vi "get TextSummary.vi"(8 "error in (no error)":errorcluster, 11 "Category in":refnum<class "Category.lvclass">) -> (0 "error out":errorcluster, 2 "Text Summary":string, 3 "Category out":refnum<class "Category.lvclass">)   [LabVIEW 2013, in "Category.lvclass"]
doc: "Text Summary is the string that appears in the second column of the tree control. It summaries the state of the xceDataNode."
uses:
  Category.lvclass
  xCE/xceDataNode/xceDataNode.lvclass
  Category.lvclass/Category.ctl
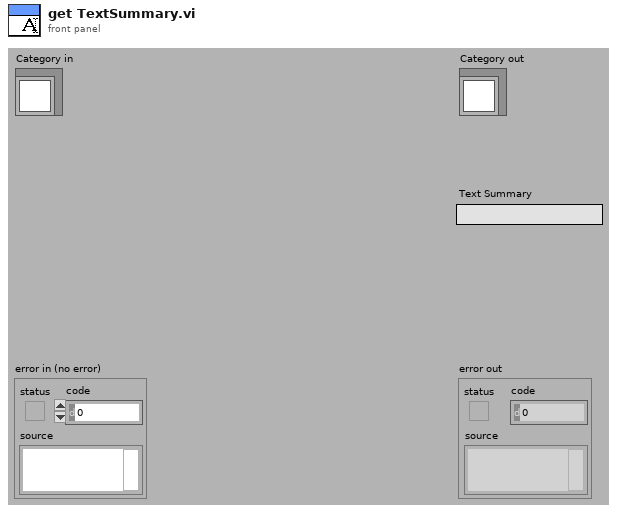
[diagram p1: front panel]
types:
  T1 = typedef "enum_Symbols.ctl" = enum16{"Default", "Analog Input", "Analog Output", "Digital Input", "Digital Output", "PWM Input", "PWM Output"}
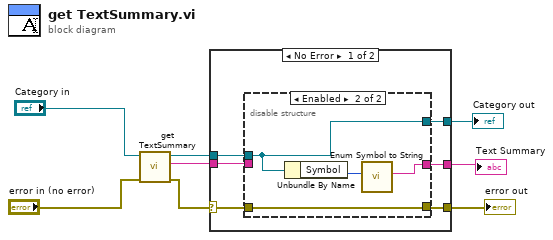
[diagram p0: block diagram]
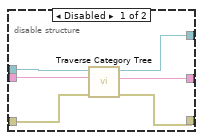
[diagram p2: hidden frame]
diagram:
  n1 = call-parent "get TextSummary.vi"("error in (no error)"="error in (no error)", "xceDataNode in"="Category in") -> ("error out"=w2:errorcluster, "Text Summary"=w1:string, "xceDataNode out"=w4:refnum<class "Category.lvclass">)  [unwired: 7 in]
  n2 = case shown="No Error" w2 {
    selector: w2 -> [w14 w27]
    tunnel: [w13 w25] -> w8
    tunnel: [w12 w26] -> w7
    tunnel: [w11 w27] -> w6
    tunnel: w4 -> [w10 w26]
    tunnel: w1 -> [w9 w25]
    frame No Error {
      n3 = disable-structure shown="Enabled" {
        disable-tunnel: w14 -> [w20 w24]
        disable-tunnel: [w19 w21] -> w13
        disable-tunnel: [w18 w23] -> w12
        disable-tunnel: [w17 w24] -> w11
        disable-tunnel: w10 -> [w16 w23]
        disable-tunnel: w9 -> [w15 _]
        frame Disabled {
          n4 = call "Traverse Category Tree.vi"("error in (no error)"=w20, "String In"=w15, "Category in"=w16) -> ("error out"=w17:errorcluster, "String Out"=w19:string, "Category out"=w18:refnum<class "Category.lvclass">)  [unwired: 6 in]
        }
        frame Enabled {
          n5 = Unbundle By Name(w23) -> ("Symbol"=w22:T1)
          n6 = call "Enum Symbol to String.vi"("Symbol Enum In"=w22) -> ("Symbol String Out"=w21:string)  [unwired: 10 in]
        }
      }
    }
    frame Error {
    }
  }
  "error out" <- w6
  "Category out" <- w7
  "Text Summary" <- w8
